vi "Main.vi"() -> ()   [LabVIEW 2015]
uses:
  TypDefs/Loop States.ctl
  TypDefs/Loop Data.ctl
panel:
  in  "device name":tag="myDAQ1"
  in  "Exit Button":bool
  in  "Start Button":bool
  out "Status":string
  in  "Clear Button":bool
  in  "Save Button":bool
  out "XY Graph":cluster{"X":dbl[], "Y":dbl[]}(graph)
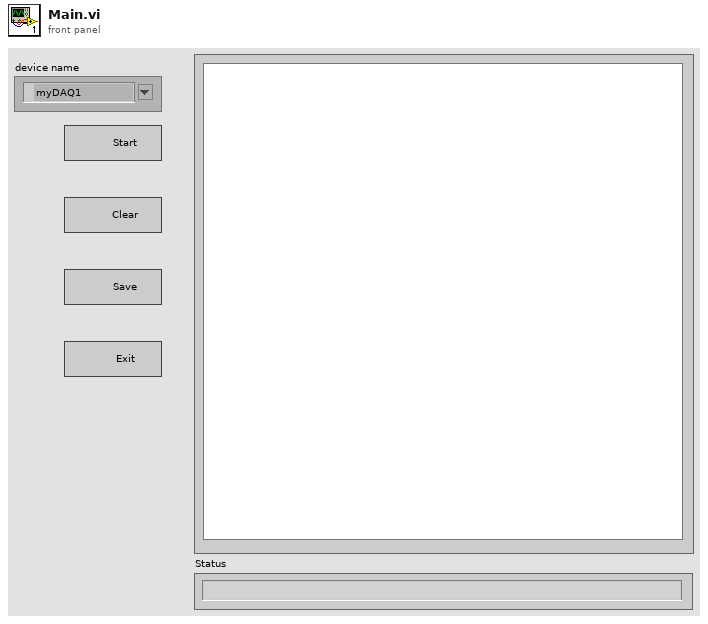
[diagram p1: front panel]
types:
  T1 = typedef "Loop Data.ctl" = cluster{"Status":string, "Graph Data":cluster{"X":dbl[], "Y":dbl[]}, "Recording Status":bool}
  T2 = typedef "Loop States.ctl" = enum16{"Error", "Wait for events", "Measure positions", "Update UI", "Initialization"}
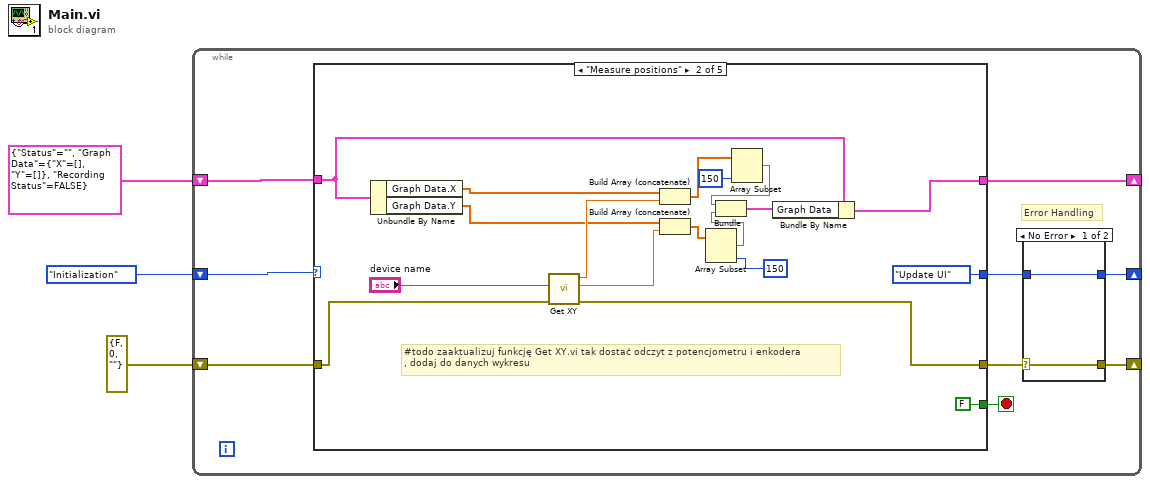
[diagram p0: block diagram]
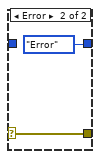
[diagram p2: hidden frame]
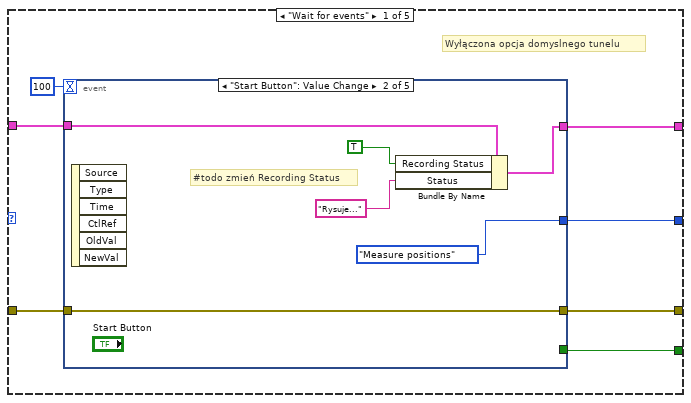
[diagram p3: hidden frame]
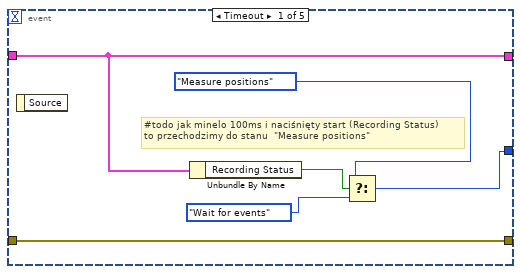
[diagram p4: hidden frame]
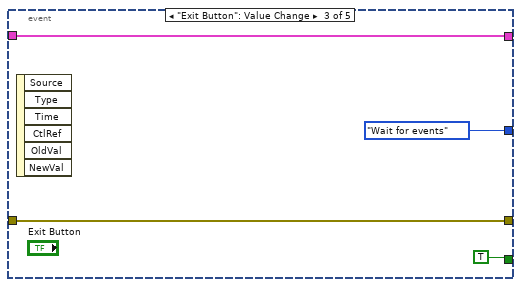
[diagram p5: hidden frame]
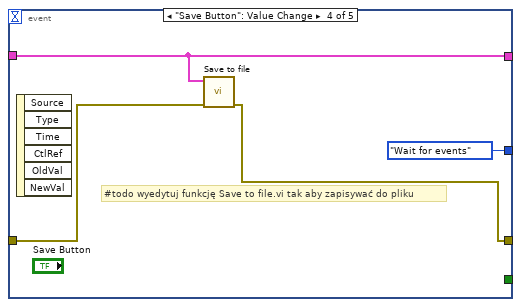
[diagram p6: hidden frame]
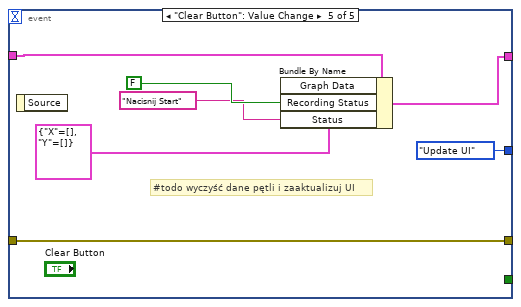
[diagram p7: hidden frame]
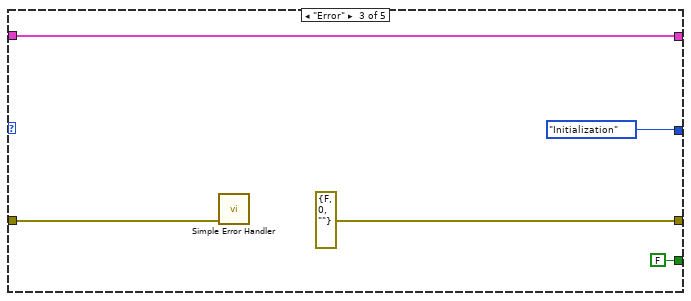
[diagram p8: hidden frame]
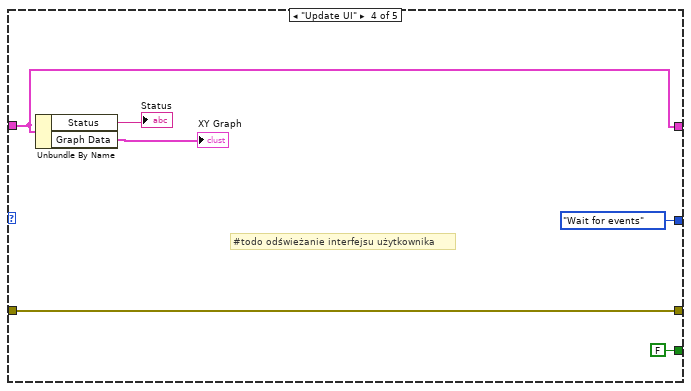
[diagram p9: hidden frame]
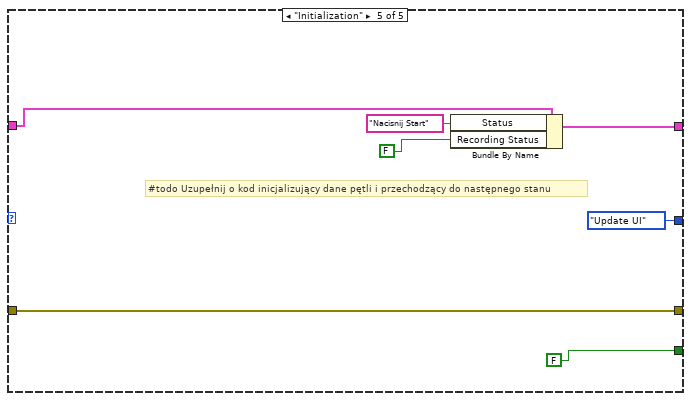
[diagram p10: hidden frame]
diagram:
  n1 = while {
    shift-right: [w10] -> _
    shift-left: T1 {"Status"="", "Graph Data"={"X"=[], "Y"=[]}, "Recording Status"=FALSE} -> [w11]
    shift-right: [w5] -> _
    shift-left: Loop_States."Initialization" -> [w12]
    shift-right: [w4] -> _
    shift-left: errorcluster {"status"=FALSE, "code"=0, "source"=""} ("error constant") -> [w8]
    stop <- w9 stop-if-true
    # "Error Handling"
    n2 = case shown="\"Measure positions\"" w12 {
      tunnel: w11 -> [w22 w65 w70 w75 w85]
      tunnel: [w20 w67 w70 w75 w84] -> w10
      tunnel: [w19 FALSE FALSE FALSE FALSE] -> w9
      tunnel: [w21 Loop_States."Update UI" Loop_States."Initialization" Loop_States."Wait for events" Loop_States."Update UI"] -> w6
      tunnel: w8 -> [w18 w64 w72 w78 w80]
      tunnel: [w17 w63 errorcluster {"status"=FALSE, "code"=0, "source"=""} ("error constant") w78 w80] -> w7
      frame "Wait for events" {
        # "Wyłączona opcja domyslnego tunelu"
        n3 = event shown="[1] \"Start Button\": Value Change" {
          selector: _ -> [_ _ _ _ _]
          dyn-events: _ -> [_ _ _ _ _]
          timeout: 100 -> [_ _ _ _ _]
          tunnel: w22 -> [w27 w33 w38 w40 w49]
          tunnel: [w24 Loop_States."Measure positions" Loop_States."Wait for events" Loop_States."Wait for events" Loop_States."Update UI"] -> w21
          tunnel: [w27 w32 w38 w40 w48] -> w20
          tunnel: [_ _ TRUE _ _] -> w19
          tunnel: w18 -> [w29 w34 w36 w42 w50]
          tunnel: [w29 w34 w36 w41 w50] -> w17
          event Timeout {
            # "#todo jak minelo 100ms i naciśnięty start (Recording Status) \nto przechodzimy do stanu  \"Measure positions\""
            n4 = event-data() -> ()  [unwired: 1 in, 1 out]
            n5 = Unbundle By Name(w27) -> ("Recording Status"=w28:bool)
            n6 = Select(t=Loop_States."Measure positions", s=w28, f=Loop_States."Wait for events") -> (s? t:f=w24:T2)
          }
          event "Start Button": Value Change {
            # "#todo zmień Recording Status"
            n7 = event-data() -> ()  [unwired: 1 in, 6 out]
            n8 = Bundle By Name(cluster=w33, "Recording Status"=TRUE, "Status"="Rysuje...") -> (w32:T1)
          }
          event "Exit Button": Value Change {
            n9 = event-data() -> ()  [unwired: 1 in, 6 out]
          }
          event "Save Button": Value Change {
            # "#todo wyedytuj funkcję Save to file.vi tak aby zapisywać do pliku"
            n10 = event-data() -> ()  [unwired: 1 in, 6 out]
            n11 = call "Save to file.vi"("error in (no error)"=w42, "Loop Data"=w40) -> ("error out"=w41:errorcluster)  [unwired: 9 in]
          }
          event "Clear Button": Value Change {
            # "#todo wyczyść dane pętli i zaaktualizuj UI"
            n12 = event-data() -> ()  [unwired: 1 in, 1 out]
            n13 = Bundle By Name(cluster=w49, "Graph Data"=cluster{"X":dbl[], "Y":dbl[]} {"X"=[], "Y"=[]}, "Recording Status"=FALSE, "Status"="Nacisnij Start") -> (w48:T1)
          }
        }
      }
      frame "Measure positions" {
        # "#todo zaaktualizuj funkcję Get XY.vi tak dostać odczyt z potencjometru i enkodera \n, dodaj do danych wykresu"
        n14 = Unbundle By Name(w65) -> ("Graph Data.X"=w59:dbl[], "Graph Data.Y"=w58:dbl[])
        n15 = call "Get XY.vi"("error in"=w64, "device name"="device name") -> ("error out"=w63:errorcluster, "Y"=w61:dbl, "X"=w60:dbl)  [unwired: 7 in]
        n16 = Build Array (concatenate)(w59, w60) -> (w54:dbl[])
        n17 = Build Array (concatenate)(w58, w61) -> (w52:dbl[])
        n18 = Array Subset(array=w52, length=150) -> (w51:dbl[])  [unwired: 1 in]
        n19 = Array Subset(array=w54, length=150) -> (w53:dbl[])  [unwired: 1 in]
        n20 = Bundle(w53, w51) -> (w56:cluster{dbl[], dbl[]})  [unwired: 1 in]
        n21 = Bundle By Name(cluster=w65, "Graph Data"=w56) -> (w67:T1)
      }
      frame "Error" {
        n22 = call <vilib>:"Simple Error Handler.vi"("error in (no error)"=w72) -> ()  [unwired: 4 in, 5 out]
      }
      frame "Update UI" {
        # "#todo odświeżanie interfejsu użytkownika"
        n23 = Unbundle By Name(w75) -> ("Status"=→"Status":string, "Graph Data"=→"XY Graph":cluster{"X":dbl[], "Y":dbl[]})
      }
      frame "Initialization" {
        # "#todo Uzupełnij o kod inicjalizujący dane pętli i przechodzący do następnego stanu"
        n24 = Bundle By Name(cluster=w85, "Status"="Nacisnij Start", "Recording Status"=FALSE) -> (w84:T1)
      }
    }
    n25 = case shown="No Error" w7 {
      selector: w7 -> [w13 w15]
      tunnel: w6 -> [w14 _]
      tunnel: [w14 Loop_States."Error"] -> w5
      tunnel: [w13 w15] -> w4
      frame No Error {
      }
      frame Error {
      }
    }
  }
